vi "Update UI Details.vi"(8 "error in":errorcluster, 9 "UI path":path, 10 "measurement service name":string, 11 "project ref":refnum<vi>) -> (0 "error out":errorcluster, 3 "project ref out":refnum<vi>)   [LabVIEW 2020, in "MeasurementService Editor.lvlib"]
uses:
  MeasurementService Editor.lvlib
  <vilib>/MeasurementLink/MeasurementLink Measurement Server/Helpers/TypeDefs/User Interface Information.ctl
  <vilib>/MeasurementLink/MeasurementLink Measurement Server/MeasurementLink Measurement Server.lvlib
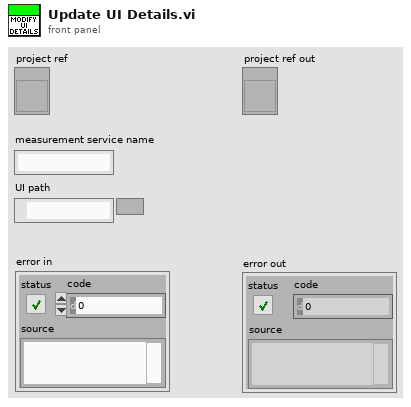
[diagram p1: front panel]
types:
  T1 = typedef "MeasurementLink Measurement Server.lvlib/User Interface Information.ctl" = cluster{"file":string}
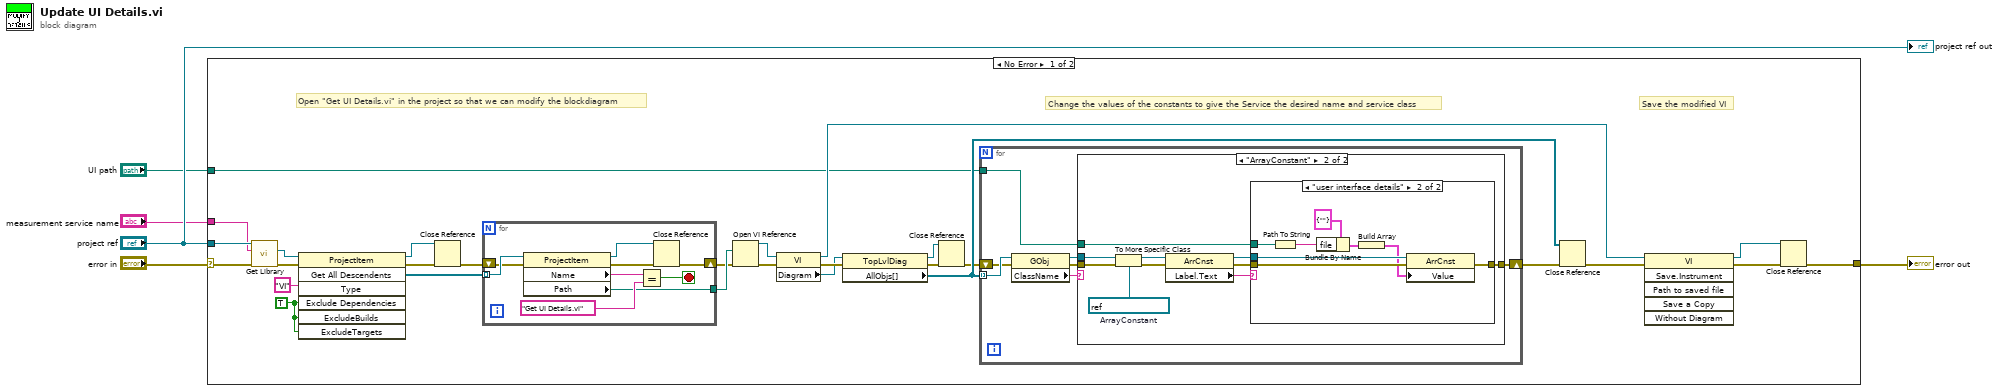
[diagram p0: block diagram]
diagram:
  n1 = case shown="No Error" "error in" {
    selector: "error in" -> [w21 w70]
    tunnel: "project ref" -> [w20 _]
    tunnel: [w31 w70] -> w3
    tunnel: "measurement service name" -> [w14 _]
    tunnel: "UI path" -> [w6 _]
    frame No Error {
      w33 = TRUE ("ExcludeDependencies")
      # "Save the modified VI"
      # "Open \"Get UI Details.vi\" in the project so that we can modify the blockdiagram"
      # "Change the values of the constants to give the Service the desired name and service class"
      n2 = call "Get Library.vi"("error in (no error)"=w21, "library name"=w14, "project ref"=w20) -> ("error out"=w19:errorcluster, "library item"=w18:refnum<vi>)  [unwired: 5 in, 2 out]
      n3 = invoke class="ProjectItem" method="Get All Descendents"(reference=w18, error in=w19, "Type"="VI", "Exclude Dependencies"=w33, "ExcludeBuilds"=w33, "ExcludeTargets"=w33) -> (reference out=w15:refnum<vi>, error out=w17:errorcluster, "All Descendents"=w13:refnum<vi>[])  [unwired: 1 in, 4 out]
      n4 = Close Reference(reference=w15, error in (no error)=w17) -> (error out=w16:errorcluster)
      n5 = for {
        tunnel: w13 -> [w69] mode=indexing
        shift-right: [w62] -> w11
        shift-left: w16 -> [w66]
        tunnel: [w64] -> w12
        stop <- w65 stop-if-true
        n6 = property class="ProjectItem"(reference=w69, error in=w66) -> (reference out=w61:refnum<vi>, error out=w63:errorcluster, "Name"=w67:string, "Path"=w64:path)
        n7 = Equal?(x=w67, y="Get UI Details.vi") -> (x = y?=w65:bool)
        n8 = Close Reference(reference=w61, error in (no error)=w63) -> (error out=w62:errorcluster)
      }
      n9 = Open VI Reference(vi path=w12, error in (no error)=w11) -> (vi reference=w28:refnum<vi>, error out=w26:errorcluster)  [unwired: 4 in]
      n10 = property class="VI"(reference=w28, error in=w26) -> (reference out=w24:refnum<vi>, error out=w27:errorcluster, "Diagram"=w25:refnum<vi>)
      n11 = property class="TopLvlDiag"(reference=w25, error in=w27) -> (reference out=w7:refnum<vi>, error out=w9:errorcluster, "AllObjs[]"=w10:refnum<vi>[])
      n12 = Close Reference(reference=w7, error in (no error)=w9) -> (error out=w8:errorcluster)
      n13 = for {
        tunnel: w10 -> [w40] mode=indexing
        shift-right: [w36] -> w23
        shift-left: w8 -> [w39]
        tunnel: w6 -> [w34]
        n14 = property class="GObj"(reference=w40, error in=w39) -> (reference out=w38:refnum<vi>, error out=w37:errorcluster, "ClassName"=w35:string)
        n15 = case shown="\"ArrayConstant\"" w35 {
          tunnel: w38 -> [_ w50]
          tunnel: w37 -> [w41 w49]
          tunnel: w34 -> [_ w48]
          tunnel: [w41 w47] -> w36
          frame Default {
          }
          frame "ArrayConstant" {
            w51 = refnum<vi> refnum  # ArrayConstant
            n16 = To More Specific Class(target class=w51, reference=w50, error in=w49) -> (specific class reference=w46:refnum<vi>, error out=w45:errorcluster)
            n17 = property class="ArrCnst"(reference=w46, error in=w45) -> (reference out=w44:refnum<vi>, error out=w43:errorcluster, "Label.Text"=w42:string)
            n18 = case shown="\"user interface details\"" w42 {
              tunnel: w48 -> [_ w54]
              tunnel: [w52 w60] -> w47
              tunnel: w44 -> [_ w59]
              tunnel: w43 -> [w52 w58]
              frame Default {
              }
              frame "user interface details" {
                n19 = Path To String(path=w54) -> (string=w53:string)
                n20 = Bundle By Name(cluster=T1 {"file"=""} ("UI Information"), "file"=w53) -> (w56:T1)
                n21 = Build Array(w56) -> (w55:T1[])
                n22 = property class="ArrCnst"(reference=w59, error in=w58, "Value"=w55) -> (error out=w60:errorcluster)  [unwired: 1 out]
              }
            }
          }
        }
      }
      n23 = Close Reference(reference=w10, error in (no error)=w23) -> (error out=w22:errorcluster)
      n24 = invoke class="VI" method="Save.Instrument"(reference=w24, error in=w22) -> (reference out=w30:refnum<vi>, error out=w29:errorcluster)  [unwired: 4 in, 4 out]
      n25 = Close Reference(reference=w30, error in (no error)=w29) -> (error out=w31:errorcluster)
    }
    frame Error {
    }
  }
  "error out" <- w3
  "project ref out" <- "project ref"
